vi "Add Command.vi"(6 "Pad":cluster{"Length":u16, "Pad Value":u16} {"Pad Value" format="%x"}, 8 "error in (no error)":errorcluster, 9 "Linkages":T2(array[cluster]) {"Linked Channel refnum" format="%.0x"}, 10 "Command":string, 11 "Message refnum in":T1=18446744073709551615 format="%.0x") -> (0 "error out":errorcluster, 2 "Command refnum out":T1=18446744073709551615 format="%.0x", 3 "Message refnum out":T1=18446744073709551615 format="%.0x")   [LabVIEW 2019, in "Scripting API.lvlib"]
uses:
  Scripting API.lvlib
  <vilib>/NI VeriStand/Custom Device API/Custom Device Item Ref.ctl
  <vilib>/NI VeriStand/Custom Device API/Custom Device API.lvlib
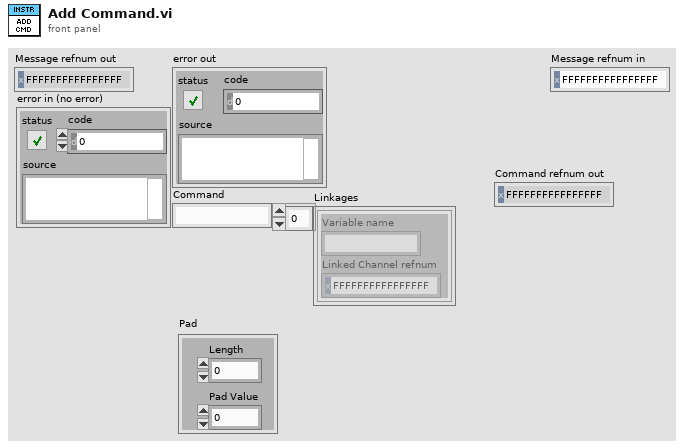
[diagram p1: front panel]
types:
  T1 = typedef "Custom Device API.lvlib/Custom Device Item Ref.ctl" = u64
  T2 = cluster{"Variable name":string, "Linked Channel refnum":T1}[]
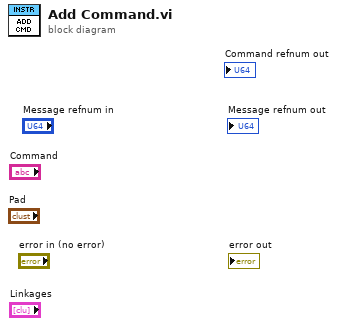
[diagram p0: block diagram]
diagram:
